vi "Log.vi"(7 "log level":T1=enum."Critical", 9 "data (null)":variant, 10 "message":string, 11 "logger in":refnum<class "Logger.lvclass">) -> (3 "logger out":refnum<class "Logger.lvclass">)   [LabVIEW 2024, in "Logging.lvlib" / "Logger.lvclass"]
uses:
  Logger.lvclass
  Log Levels.ctl
  Internal Log Levels.ctl
  Logger.lvclass/Logger.ctl
  Filters/Scopes/Scope/Scope.lvclass
  Filters/Filter/Filter.lvclass
  Logging.lvlib
panel:
  # "Connector Pane"
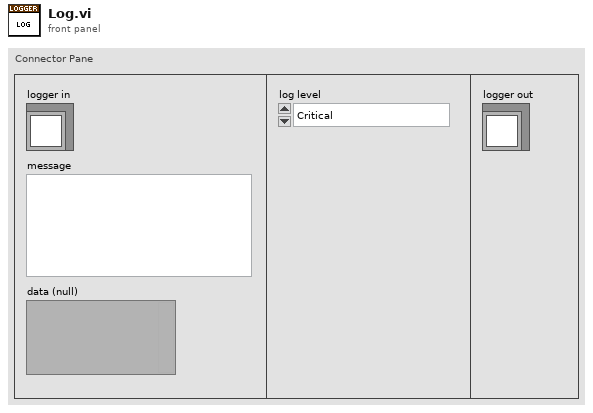
[diagram p1: front panel]
types:
  T1 = typedef "Logging.lvlib/Log Levels.ctl" = enum16{"Trace", "Debug", "Info", "Warning", "Error", "Critical"}
  T2 = typedef "Logging.lvlib/Internal Log Levels.ctl" = enum16{"Trace", "Debug", "Info", "Warning", "Error", "Critical", "Internal"}
  T3 = typedef "Logging.lvlib/Log Record.ctl" = cluster{"level":T2, "timestamp":timestamp, "call chain":string[], "message":string, "data":variant}
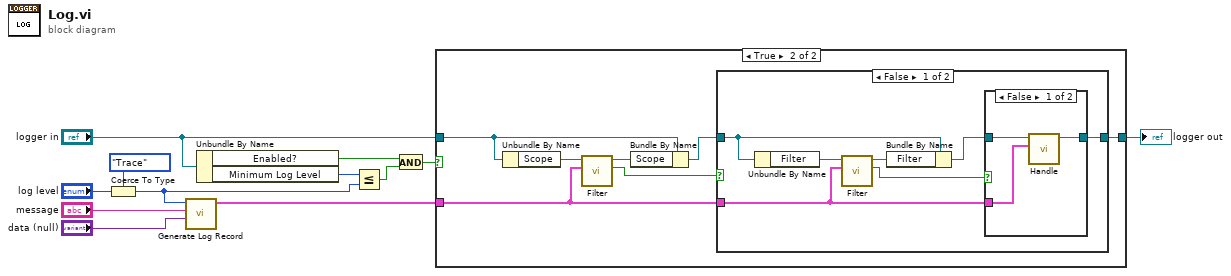
[diagram p0: block diagram]
diagram:
  n1 = Coerce To Type(0:"log level", 1:Internal_Log_Levels."Trace" ("internal log level")) -> (2:w2:T2)
  n2 = call "Generate Log Record.vi"("data (null)"="data (null)", "message (\"\")"="message", "level (Internal)"=w2) -> ("log record"=w3:T3)  [unwired: 8 in]
  n3 = Unbundle By Name("logger in") -> ("Enabled?"=w10:bool, "Minimum Log Level"=w9:T1)
  n4 = Less Or Equal?(x=w9, y=w2) -> (x <= y?=w8:bool)
  n5 = And(x=w10, y=w8) -> (x .and. y?=w11:bool)
  n6 = case shown="True" w11 {
    tunnel: [w13 w17] -> w6
    tunnel: w3 -> [_ w14]
    tunnel: "logger in" -> [w13 w16]
    frame False {
    }
    frame True {
      n7 = Unbundle By Name(w16) -> ("Scope"=w20:refnum<class "Scope.lvclass">)
      n8 = call-dynamic "Filter.vi"("log record"=w14, "filter in"=w20) -> ("discard?"=w15:bool, "filter out"=w19:refnum<class "Scope.lvclass">)  [unwired: 8 in]
      n9 = Bundle By Name(cluster=w16, "Scope"=w19) -> (w18:refnum<class "Logger.lvclass">)
      n10 = case shown="False" w15 {
        tunnel: w18 -> [w27 w32]
        tunnel: [w23 w32] -> w17
        tunnel: w14 -> [w22 _]
        frame False {
          n11 = Unbundle By Name(w27) -> ("Filter"=w26:refnum<class "Filter.lvclass">)
          n12 = call-dynamic "Filter.vi"("log record"=w22, "filter in"=w26) -> ("discard?"=w21:bool, "filter out"=w25:refnum<class "Filter.lvclass">)  [unwired: 8 in]
          n13 = Bundle By Name(cluster=w27, "Filter"=w25) -> (w24:refnum<class "Logger.lvclass">)
          n14 = case shown="False" w21 {
            tunnel: w24 -> [w28 w31]
            tunnel: [w30 w31] -> w23
            tunnel: w22 -> [w29 _]
            frame False {
              n15 = call "Handle.vi"("log record"=w29, "logger in"=w28) -> ("logger out"=w30:refnum<class "Logger.lvclass">)  [unwired: 9 in]
            }
            frame True {
            }
          }
        }
        frame True {
        }
      }
    }
  }
  "logger out" <- w6
